vi "Remove Previous Configurations by Name.vi"(8 "error in (no error)":errorcluster, 10 "Imported Names":string[](array[string]), 11 "Node In":u64) -> (0 "error out":errorcluster, 3 "Node Out":T1 format="%.0x")   [LabVIEW 2019, in "Diagnostics Addon System Explorer.lvlib"]
uses:
  Diagnostics Addon System Explorer.lvlib
  <vilib>/NI VeriStand/Custom Device API/Custom Device Item Ref.ctl
  <vilib>/NI VeriStand/Custom Device API/Custom Device API.lvlib
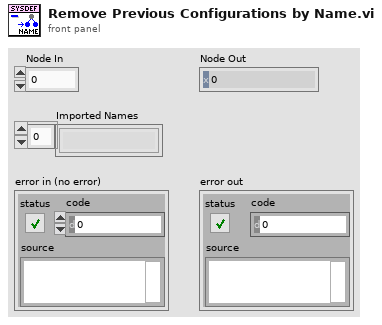
[diagram p1: front panel]
types:
  T1 = typedef "Custom Device API.lvlib/Custom Device Item Ref.ctl" = u64
  T2 = typedef "Custom Device API.lvlib/Custom Device Item Info.ctl" = cluster{"Name":string, "Is Channel":bool, "GUID":string, "Is Waveform":bool}
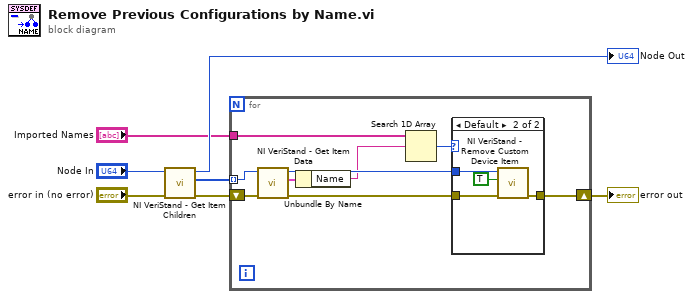
[diagram p0: block diagram]
diagram:
  n1 = call <vilib>:"NI VeriStand - Get Item Children.vi"("error in (no error)"="error in (no error)", "Item Ref in"="Node In") -> ("error out"=w1:errorcluster, "Child Refs"=w2:T1[], "Item Ref out"=→"Node Out":T1)  [unwired: 6 in, 1 out]
  n2 = for {
    shift-right: [w11] -> w6
    shift-left: w1 -> [w15]
    tunnel: w2 -> [w14] mode=indexing
    tunnel: "Imported Names" -> [w13]
    n3 = call <vilib>:"NI VeriStand - Get Item Data.vi"("error in (no error)"=w15, "Item Ref in"=w14) -> ("error out"=w12:errorcluster, "Item Info"=w16:T2, "Item Ref out"=w10:T1)  [unwired: 7 out]
    n4 = Unbundle By Name(w16) -> ("Name"=w8:string)
    n5 = Search 1D Array(1D array=w13, element=w8) -> (index of element=w9:i32)  [unwired: 1 in]
    n6 = case shown="Default" w9 {
      tunnel: w12 -> [w17 w21]
      tunnel: [w17 w20] -> w11
      tunnel: w10 -> [_ w19]
      frame -1 {
      }
      frame Default {
        n7 = call <vilib>:"NI VeriStand - Remove Custom Device Item.vi"("error in (no error)"=w21, "Force Delete (F)"=TRUE, "Item Ref in"=w19) -> ("error out"=w20:errorcluster)  [unwired: 7 in, 1 out]
      }
    }
  }
  "error out" <- w6
